vi "Create New VI Reference Control.vi"(8 "error in (no error)":errorcluster, 9 "Picture Control Ref":refnum<vi>, 10 "Path Control Ref":refnum<vi>) -> (0 "error out":errorcluster, 3 "VI Reference Control out":refnum<class "VI Reference Control.lvclass">)   [LabVIEW 2016, in "VI Reference Control.lvclass"]
uses:
  VI Reference Control.lvclass
  C:/Users/tblair/Documents/Git Projects/Drag and Drop VI Tool/Reference Control/Reference Control.lvclass
  Reference Control/Reference Control.lvclass
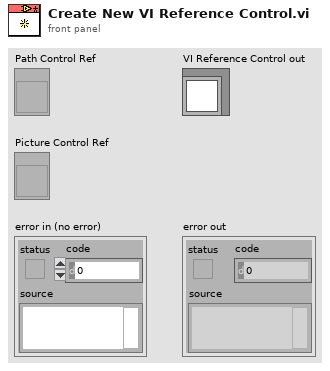
[diagram p1: front panel]
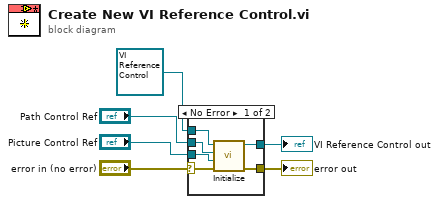
[diagram p0: block diagram]
diagram:
  n1 = case shown="No Error" "error in (no error)" {
    selector: "error in (no error)" -> [w8 w14]
    tunnel: [w7 w14] -> w5
    tunnel: [w12 w13] -> w3
    tunnel: refnum<class "VI Reference Control.lvclass"> refnum ("VI Reference Control in") -> [w11 w13]
    tunnel: "Path Control Ref" -> [w10 _]
    tunnel: "Picture Control Ref" -> [w9 _]
    frame No Error {
      n2 = call "Initialize.vi"("error in (no error)"=w8, "Picture Control Ref"=w9, "Path Control Ref"=w10, "Reference Control in"=w11) -> ("error out"=w7:errorcluster, "Reference Control out"=w12:refnum<class "VI Reference Control.lvclass">)  [unwired: 6 in]
    }
    frame Error {
    }
  }
  "error out" <- w5
  "VI Reference Control out" <- w3
